vi "MindwaveCompute2Bytes.vi"(1 "INDEX":u8, 2 "RAW_ARRAY":u8[](array[numeric]) format="%x") -> (0 "RAW_VALUE":i16 format="%x")   [LabVIEW 2011, in "Neurosky.lvlib"]
uses:
  Users/Isaias/Documents/GitHub/Neurosky/Neurosky.lvlib
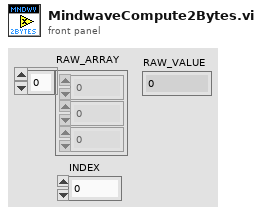
[diagram p1: front panel]
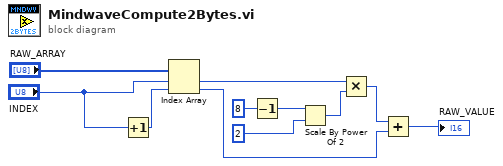
[diagram p0: block diagram]
diagram:
  n1 = Increment(x="INDEX") -> (x+1=w10:u8)
  n2 = Index Array(array="RAW_ARRAY", index #1="INDEX", index #2=w10) -> (element #1=w5:u8, element #2=w2:u8)
  n3 = Decrement(x=u8 8 ("y")) -> (x-1=w7:u8)
  n4 = Scale By Power Of 2(n=w7, x=u16 2 ("y")) -> (x*2^n=w4:u16)
  n5 = Multiply(x=w5, y=w4) -> (x*y=w3:u16)
  n6 = Add(x=w3, y=w2) -> (x+y=→"RAW_VALUE":u16)
